vi "Vision Research Phantom Series PhCon PhSetSingleCineParams.vi"(0 "CN in":u32=1, 3 "ACQUIPARAMS":T1 {"CFA"."CFA" items=["CFA_NONE", "CFA_VRI", "CFA_VRIV6", "CFA_BAYER", "CFA_BAYERFLIP"]; "TriggerTime"."fractions" format="%32.0f"}, 5 "Error In (no error)":errorcluster) -> (14 "CN out":u32=1, 17 "ACQUIPARAMS out":T1 {"CFA"."CFA" items=["CFA_NONE", "CFA_VRI", "CFA_VRIV6", "CFA_BAYER", "CFA_BAYERFLIP"]; "TriggerTime"."fractions" format="%32.0f"}, 19 "Error Out":errorcluster)   [LabVIEW 2013, in "VRI.lvlib"]
doc: "PhSetSingleCineParams\nHRESULT PhSetSingleCineParams(UINT CN, PACQUIPARAMS pCP)\n\nParameters Description\nCN (in) Camera number,\npCP (in) Acquisition parameters to set.\nReturn HRESULT (0 = Ok)\nComments This is the reccomended way to set the acquisition\n parameters in single cine mode. You can read the last\n parameters you have set by calling the \n PhGetCineParams from CINE_PREVIEW.\n The parameters are written always to CINE_PREVIEW\n and are written to CINE_FIRST too only if\n CINE_FIRST is not already recorded."
uses:
  VRI.lvlib
  _Type Defs/PHCon ACQUIPARAMS.ctl
  _Type Defs/PhCon SyncImaging.ctl
  _Type Defs/Rect.ctl
  _Type Defs/PHCon Time64.ctl
  _Type Defs/PhInt CFA.ctl
  Phantom DLLs/PhCon.dll
panel:
  # "For instructions on the use of this VI, press Ctrl+H to display the help window and move the mouse over the icon, controls, and indicators"
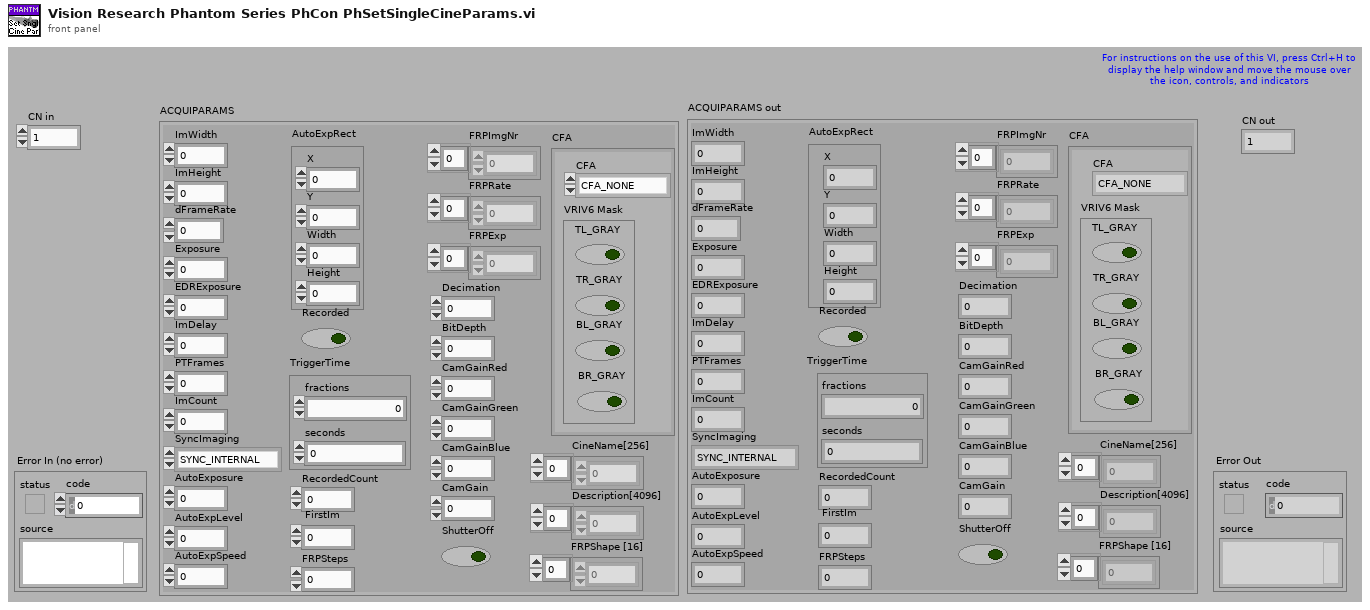
[diagram p1: front panel]
types:
  T1 = typedef "VRI.lvlib/PHCon ACQUIPARAMS.ctl" = cluster{"ImWidth":u32, "ImHeight":u32, "(deprecated)FrameRateInt":u32, "Exposure":u32, "EDRExposure":u32, "ImDelay":u32, "PTFrames":u32, "ImCount":u32, "SyncImaging":T2, "AutoExposure":u32, "AutoExpLevel":u32, "AutoExpSpeed":u32, "AutoExpRect":T3, "Recorded":bool, "TriggerTime":T4, "RecordedCount":u32, "FirstIm":i32, "FRPSteps":u32, "FRPImgNr":i32[], "FRPRate":u32[], "FRPExp":u32[], "Decimation":u32, "BitDepth":u32, "CamGainRed":u32, "CamGainGreen":u32, "CamGainBlue":u32, "CamGain":u32, "ShutterOff":bool, "CFA":T5, "CineName[256]":u8[], "Description[4096]":u8[], "FRPShape [16]":u32[], "dFrameRate":dbl}
  T2 = typedef "VRI.lvlib/PhCon SyncImaging.ctl" = enum32{"SYNC_INTERNAL", "SYNC_EXTERNAL", "SYNC_LOCKTOIRIG"}
  T3 = typedef "VRI.lvlib/Rect.ctl" = cluster{"X":i32, "Y":i32, "Width":i32, "Height":i32}
  T4 = typedef "VRI.lvlib/PHCon Time64.ctl" = cluster{"fractions":u32, "seconds":u32}
  T5 = typedef "VRI.lvlib/PhInt CFA.ctl" = cluster{"CFA":u32, "VRIV6 Mask":cluster{"TL_GRAY":bool, "TR_GRAY":bool, "BL_GRAY":bool, "BR_GRAY":bool}}
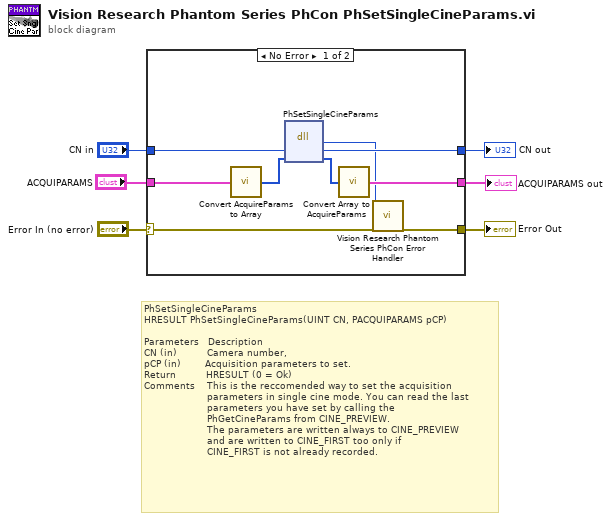
[diagram p0: block diagram]
diagram:
  # "PhSetSingleCineParams\nHRESULT PhSetSingleCineParams(UINT CN, PACQUIPARAMS pCP)\n\nParameters   Description\nCN (in)          Camera number,\npCP (in)        Acquisition parameters to set.\nReturn          HRESULT (0 = Ok)\nComments    This is the reccomended way to set the acquisition\n                     parameters in single cine mode. You can read the last\n                     parameters you have set by calling the \n                     PhGetCineParams from CINE_PREVIEW.\n                     The parameters are written always to CINE_PREVIEW\n                     and are written to CINE_FIRST too only if\n                     CINE_FIRST is not already recorded."
  n1 = case shown="No Error" "Error In (no error)" {
    selector: "Error In (no error)" -> [w15 w17]
    tunnel: [w14 w17] -> w5
    tunnel: "CN in" -> [w13 w16]
    tunnel: [w12 w16] -> w3
    tunnel: "ACQUIPARAMS" -> [w11 _]
    tunnel: [w10 _] -> w1
    frame No Error {
      n2 = call "Convert AcquireParams to Array.vi"("ACQUIPARAMS"=w11) -> ("ACQUIPARAMS Data Array"=w8:u32[])
      n3 = dll-call lib="C:/Projects/SDK/32-bit/Vision Research Phantom Series Labview Driver/Phantom DLLs/PhCon.dll" fn="PhSetSingleCineParams"("CN"=w13, "pCP"=w8) -> ("HRESULT"=w9:i32, "CN"=w12:u32, "pCP"=w7:u32[])  [unwired: 3 in, 2 out]
      n4 = call "Convert Array to AcquireParams.vi"("ACQUIPARAMS BYTE ARRAY"=w7) -> ("ACQUIPARAMS"=w10:T1)
      n5 = call "Vision Research Phantom Series PhCon Error Handler.vi"("ErrNo"=w9, "Error In (no error)"=w15) -> ("Error Out"=w14:errorcluster)  [unwired: 17 out]
    }
    frame Error {
    }
  }
  "Error Out" <- w5
  "CN out" <- w3
  "ACQUIPARAMS out" <- w1
